vi "MbusRegDataConvert.vi"() -> ()   [LabVIEW 2019]
panel:
  out "(hi.lo)":u16
  out "element 2":u8
  out "element":u8
  out "unsigned byte array":u8[](array[numeric])
  out "*(type *) &x 10":i32
  out "*(type *) &x 9":i32
  out "Array":i32[](array[numeric])
  in  "*(type *) &x 8":string
  out "*(type *) &x 7":i32
  in  "*(type *) &x 6":string
  out "*(type *) &x 5":i32
  out "*(type *) &x 4":i32
  out "*(type *) &x 3":string
  out "*(type *) &x 2":i32
  out "*(type *) &x":string
  out "hex integer string":string
  out "String":string
  out "appended array":u8[](array[numeric])
  out "hi(x) 2":u8
  out "lo(x) 2":u8
  out "lo(x)":u8
  out "hi(x)":u8
  out "string":string
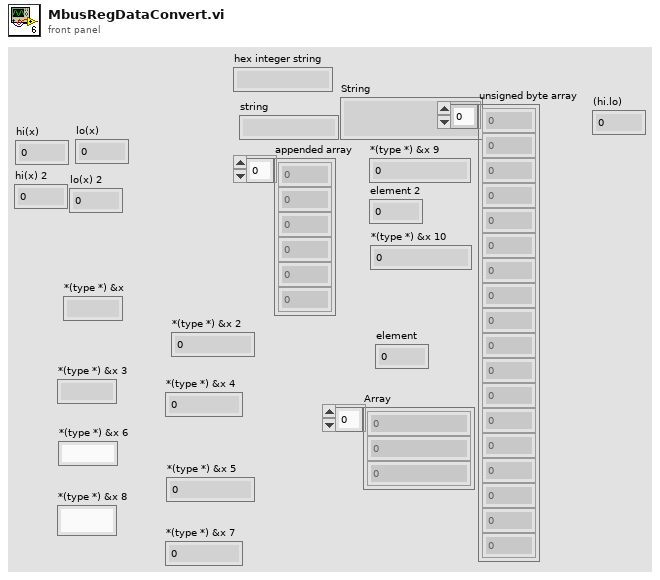
[diagram p1: front panel]
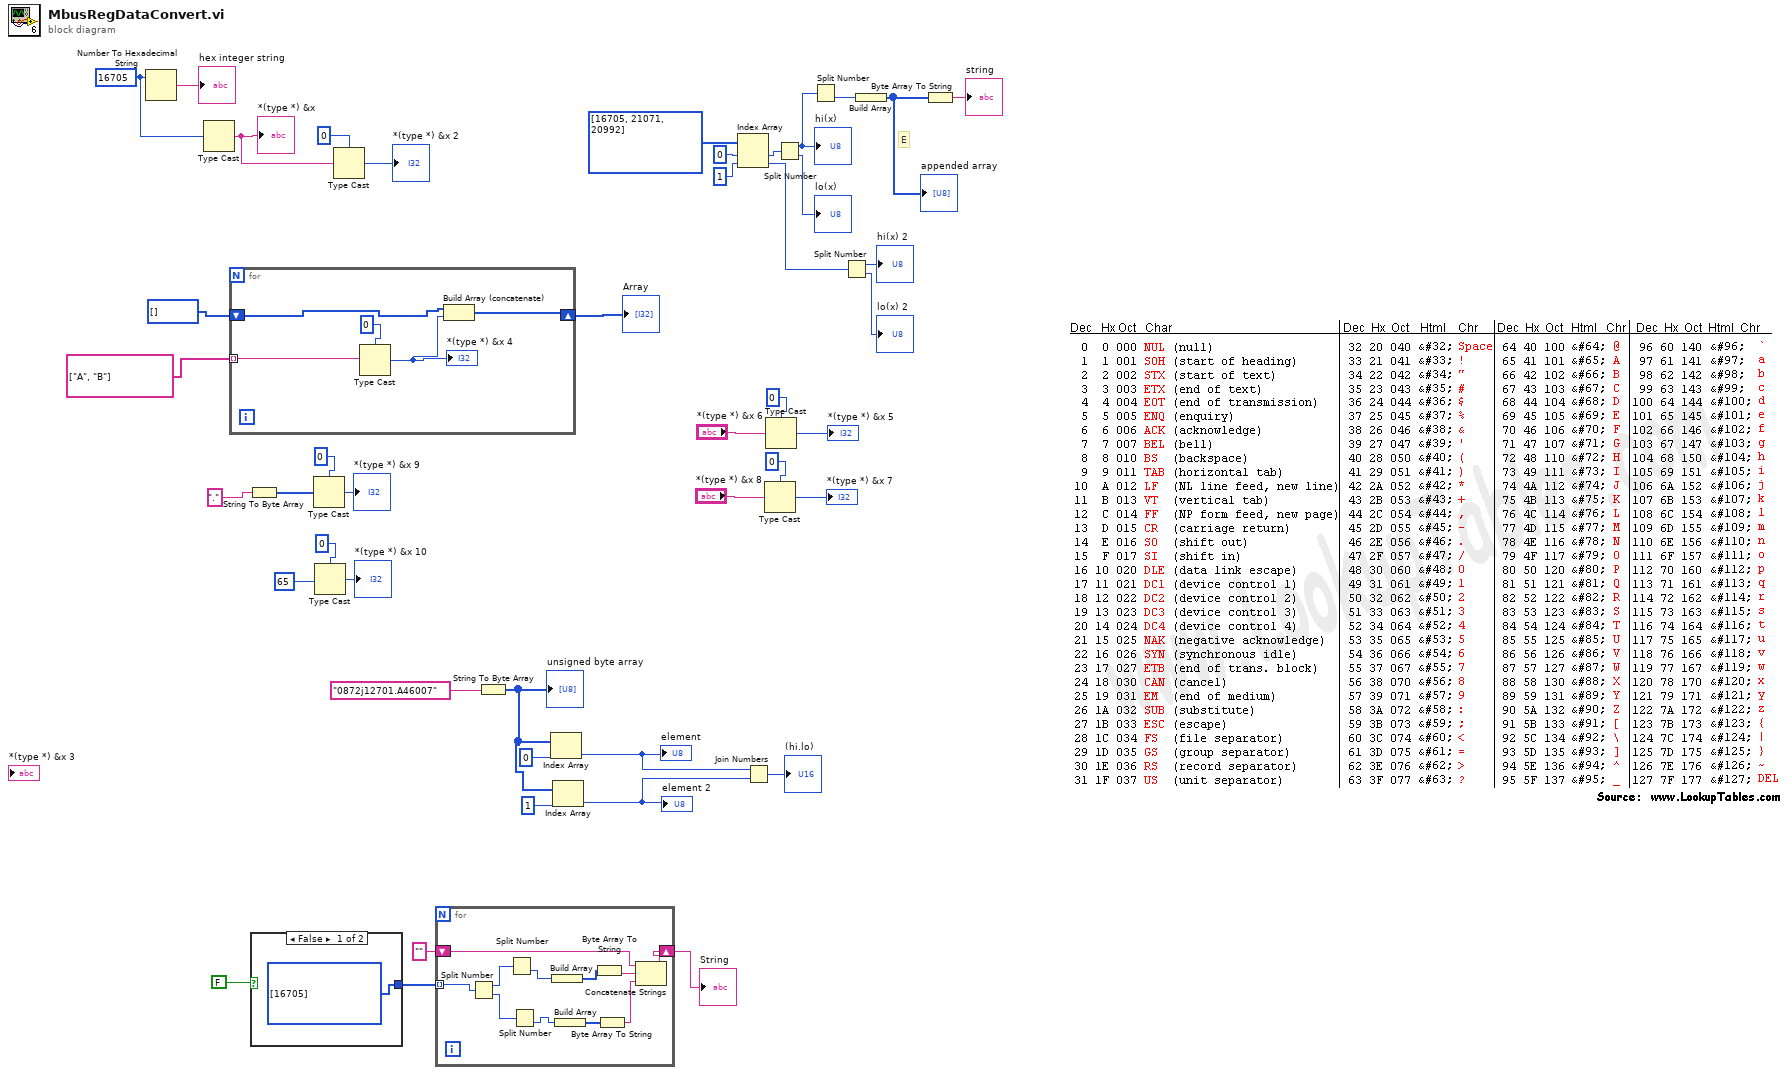
[diagram p0: block diagram]
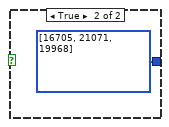
[diagram p2: hidden frame]
diagram:
  w27 = 16705 ("number")
  # "E"
  n1 = Number To Hexadecimal String(2:w27) -> (0:→"hex integer string":string)  [unwired: 1 in]
  n2 = Type Cast(x=w27) -> (*(type *) &x=w25:string)  [unwired: 1 in]
  "*(type *) &x" <- w25
  n3 = for {
    tunnel: string[] ["A", "B"] -> [w48] mode=indexing
    shift-right: [w45] -> w15
    shift-left: i32[] [] -> [w47]
    n4 = Type Cast(type=0, x=w48) -> (*(type *) &x=w46:i32)
    "*(type *) &x 4" <- w46
    n5 = Build Array (concatenate)(w47, w46) -> (w45:i32[])
  }
  "Array" <- w15
  n6 = String To Byte Array(string=".") -> (unsigned byte array=w13:u8[])
  n7 = case shown="False" FALSE {
    tunnel: [u16[] [16705] ("unsigned byte array") u16[] [16705, 21071, 19968] ("unsigned byte array")] -> w32
    frame False {
    }
    frame True {
    }
  }
  n8 = Type Cast(type=0, x=w13) -> (*(type *) &x=→"*(type *) &x 9":i32)
  n9 = Type Cast(type=0, x=65) -> (*(type *) &x=→"*(type *) &x 10":i32)
  n10 = Type Cast(type=0, x=w25) -> (*(type *) &x=→"*(type *) &x 2":i32)
  n11 = for {
    tunnel: w32 -> [w62] mode=indexing
    shift-right: [w54] -> w30
    shift-left: "" -> [w55]
    n12 = Split Number(x=w62) -> (hi(x)=w60:u8, lo(x)=w58:u8)
    n13 = Split Number(x=w60) -> (lo(x)=w53:u8)  [unwired: 1 out]
    n14 = Split Number(x=w58) -> (lo(x)=w52:u8)  [unwired: 1 out]
    n15 = Build Array(w53) -> (w61:u8[])
    n16 = Build Array(w52) -> (w59:u8[])
    n17 = Byte Array To String(unsigned byte array=w61) -> (string=w57:string)
    n18 = Byte Array To String(unsigned byte array=w59) -> (string=w56:string)
    n19 = Concatenate Strings(w55, w57, w56) -> (w54:string)
  }
  "String" <- w30
  n20 = String To Byte Array(string="0872j12701.A46007") -> (unsigned byte array=w4:u8[])
  "unsigned byte array" <- w4
  n21 = Index Array(array=w4, index=0) -> (element=w3:u8)
  "element" <- w3
  n22 = Index Array(array=w4, index=1) -> (element=w2:u8)
  "element 2" <- w2
  n23 = Index Array(array=u16[] [16705, 21071, 20992] ("unsigned byte array"), index #1=0 ("index"), index #2=1 ("index")) -> (element #1=w43:u16, element #2=w39:u16)
  n24 = Join Numbers(hi=w3, lo=w2) -> ((hi.lo)=→"(hi.lo)":u16)
  n25 = Type Cast(type=0, x="*(type *) &x 8") -> (*(type *) &x=→"*(type *) &x 7":i32)
  n26 = Type Cast(type=0, x="*(type *) &x 6") -> (*(type *) &x=→"*(type *) &x 5":i32)
  n27 = Split Number(x=w43) -> (hi(x)=w36:u8, lo(x)=→"lo(x)":u8)
  "hi(x)" <- w36
  n28 = Split Number(x=w36) -> (lo(x)=w33:u8)  [unwired: 1 out]
  n29 = Split Number(x=w39) -> (hi(x)=→"hi(x) 2":u8, lo(x)=→"lo(x) 2":u8)
  n30 = Build Array(w33) -> (w34:u8[])
  "appended array" <- w34
  n31 = Byte Array To String(unsigned byte array=w34) -> (string=→"string":string)
